vi "Base64Decoder.vi"(11 "String In":string) -> (1 "Base64ByteArray":u8[](array[numeric]) format="%b", 3 "String Out":string)   [LabVIEW 2009]
doc: "Decode a base64 encoded string into a binary string"
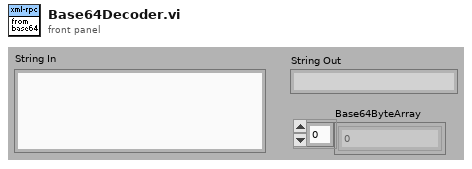
[diagram p1: front panel]
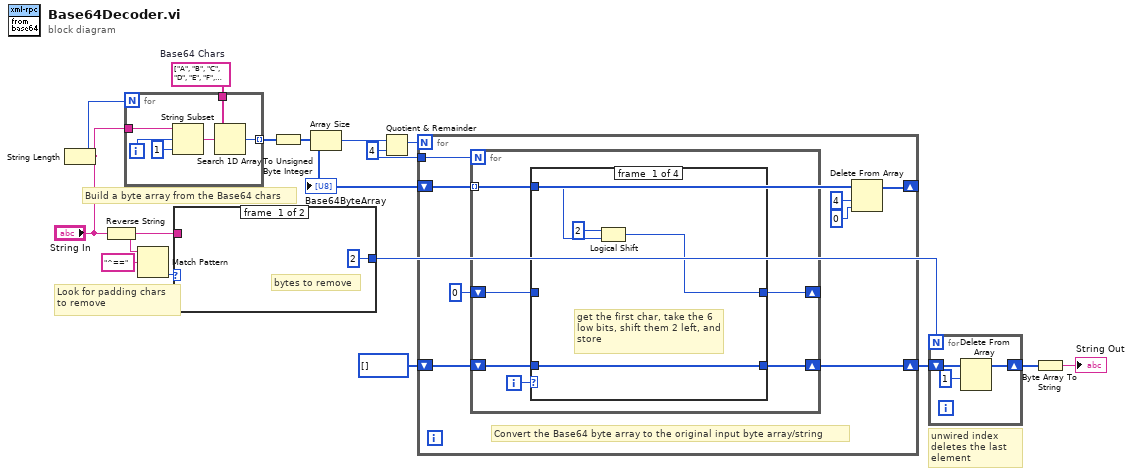
[diagram p0: block diagram]
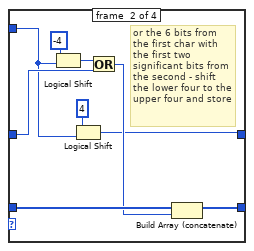
[diagram p2: hidden frame]
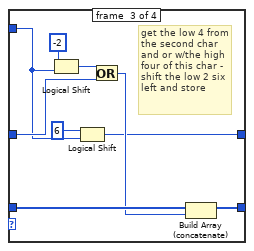
[diagram p3: hidden frame]
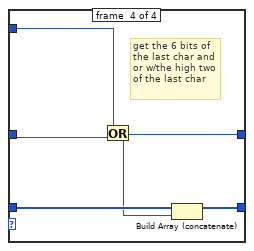
[diagram p4: hidden frame]
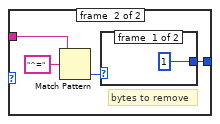
[diagram p5: hidden frame]
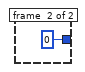
[diagram p6: hidden frame]
diagram:
  w6 = string[] ["A", "B", "C", "D", "E", "F", "G", "H", "I", "J", "K", "L", "M", "N", "O", "P", "Q", "R", "S", "T", "U", "V", "W", "X", "Y", "Z", "a", "b", "c", "d", "e", "f", "g", "h", "i", "j", "k", "l", "m", "n", "o", "p", "q", "r", "s", "t", "u", "v", "w", "x", "y", "z", "0", "1", "2", "3", "4", "5", "6", "7", "8", "9", "+", "/"]  # Base64 Chars
  w12 = 4 ("y")
  # "unwired index deletes the last element"
  # "Build a byte array from the Base64 chars"
  # "Look for padding chars\nto remove"
  n1 = String Length(string="String In") -> (length=w8:i32)
  n2 = Reverse String(1:"String In") -> (0:w14:string)
  n3 = for {
    N: w8 -> [_]
    tunnel: "String In" -> [w20]
    tunnel: w6 -> [w19]
    tunnel: [w17] -> w5 mode=indexing
    i -> [w22]
    n4 = String Subset(string=w20, offset (0)=w22, length (rest)=1 ("length (rest)")) -> (substring=w18:string)
    n5 = Search 1D Array(1D array=w19, element=w18) -> (index of element=w17:i32)  [unwired: 1 in]
  }
  n6 = Match Pattern(string=w14, regular expression="^==") -> (offset past match=w15:i32)  [unwired: 1 in, 3 out]
  n7 = case shown="-1" w15 {
    tunnel: [2 w25] -> w1
    tunnel: w14 -> [_ w24]
    frame #0 {
      # "bytes to remove"
    }
    frame #1 {
      # "bytes to remove"
      n8 = Match Pattern(string=w24, regular expression="^=") -> (offset past match=w26:i32)  [unwired: 1 in, 3 out]
      n9 = case shown="-1" w26 {
        tunnel: [1 0] -> w25
        frame #0 {
        }
        frame #1 {
        }
      }
    }
  }
  n10 = To Unsigned Byte Integer(number=w5) -> (unsigned 8bit integer=w4:u8[])
  "Base64ByteArray" <- w4
  n11 = Array Size(array=w4) -> (size(s)=w13:i32)
  n12 = Quotient & Remainder(x=w13, y=w12) -> (floor(x/y)=w9:i32)  [unwired: 1 out]
  n13 = for {
    N: w9 -> [_]
    tunnel: w12 -> [w37]
    shift-right: [w33] -> _
    shift-left: w4 -> [w36]
    shift-right: [w31] -> w3
    shift-left: u8[] [] ("Base64ByteArray") -> [w32]
    # "Convert the Base64 byte array to the original input byte array/string"
    n14 = for {
      N: w37 -> [_]
      tunnel: w36 -> [w43] mode=indexing
      shift-right: [w42] -> _
      shift-left: u8 0 -> [w40]
      shift-right: [w38] -> w31
      shift-left: w32 -> [w39]
      i -> [w41]
      n15 = case shown="2" w41 {
        tunnel: w43 -> [w47 w50 w57 w70]
        tunnel: [w45 w48 w58 w67] -> w42
        tunnel: w40 -> [_ w54 w60 w69]
        tunnel: w39 -> [w44 w53 w63 w68]
        tunnel: [w44 w52 w61 w66] -> w38
        frame #0 {
          # "get the first char, take the 6 low bits, shift them 2 left, and store"
          n16 = Logical Shift(y=i8 2, x=w47) -> (x << y=w45:u8)
        }
        frame #1 {
          # "or the 6 bits from the first char with the first two significant bits from the second - shift the lower four to the upper four and store"
          n17 = Logical Shift(y=i8 -4, x=w50) -> (x << y=w55:u8)
          n18 = Logical Shift(y=i8 4, x=w50) -> (x << y=w48:u8)
          n19 = Or(x=w55, y=w54) -> (x .or. y?=w51:u8)
          n20 = Build Array (concatenate)(w53, w51) -> (w52:u8[])
        }
        frame #2 {
          # "get the low 4 from the second char and or w/the high four of this char - shift the low 2 six left and store"
          n21 = Logical Shift(y=i8 -2, x=w57) -> (x << y=w64:u8)
          n22 = Logical Shift(y=u8 6, x=w57) -> (x << y=w58:u8)
          n23 = Or(x=w64, y=w60) -> (x .or. y?=w62:u8)
          n24 = Build Array (concatenate)(w63, w62) -> (w61:u8[])
        }
        frame #3 {
          # "get the 6 bits of the last char and or w/the high two of the last char"
          n25 = Or(x=w70, y=w69) -> (x .or. y?=w67:u8)
          n26 = Build Array (concatenate)(w68, w67) -> (w66:u8[])
        }
      }
    }
    n27 = Delete From Array(array=w36, length=4, index=0) -> (array with subset deleted=w33:u8[])  [unwired: 1 out]
  }
  n28 = for {
    N: w1 -> [_]
    shift-right: [w72] -> w2
    shift-left: w3 -> [w73]
    n29 = Delete From Array(array=w73, length=1) -> (array with subset deleted=w72:u8[])  [unwired: 1 in, 1 out]
  }
  n30 = Byte Array To String(unsigned byte array=w2) -> (string=→"String Out":string)
